vi "Elevator2.vi"() -> ()   [LabVIEW 2020]
uses:
  meter.ctl
  States.ctl
  <vilib>/MakerHub/LINX/Public/Peripherals/Digital/Digital Read N Chans.vi
  <vilib>/MakerHub/LINX/Private/Local IO/LinxDigitalRead.vi
  <vilib>/MakerHub/LINX/Public/Utilities/Check Channel.vi
  <vilib>/MakerHub/LINX/Public/Utilities/Open Serial.vi
  <vilib>/MakerHub/LINX/Private/Utilties/Generate Error.vi
  <vilib>/MakerHub/LINX/LMH-LINX.lvlib
panel:
  in  "Floor 1":bool
  in  "Floor 2":bool
  in  "Floor 3":bool
  in  "Floor 4":bool
  in  "DI Channels":u8[](array[numeric])
  in  "Serial Port":refnum<visa-resource-name>="N/A"
  in  "Run time error":errorcluster
  out "Arrow":u16(ring)
  out "Meter 1":T1 scale=1.0..4.0
  out "Meter 2":T1 scale=1.0..4.0
  out "Meter 4":T1 scale=1.0..4.0
  out "Meter 3":T1 scale=1.0..4.0
  in  "Down (2)":bool
  in  "Up (1)":bool
  in  "Up (2)":bool
  in  "Up (3)":bool
  in  "Down (3)":bool
  in  "Down (4)":bool
  out "Ring 1":u16(ring)
  out "Ring 2":u16(ring)
  out "Ring 3":u16(ring)
  out "Ring 4":u16(ring)
  out "Slider":dbl(slide) step=1.0 scale=1.0..4.0
  out "Floor #":u8
  in  "stop":bool
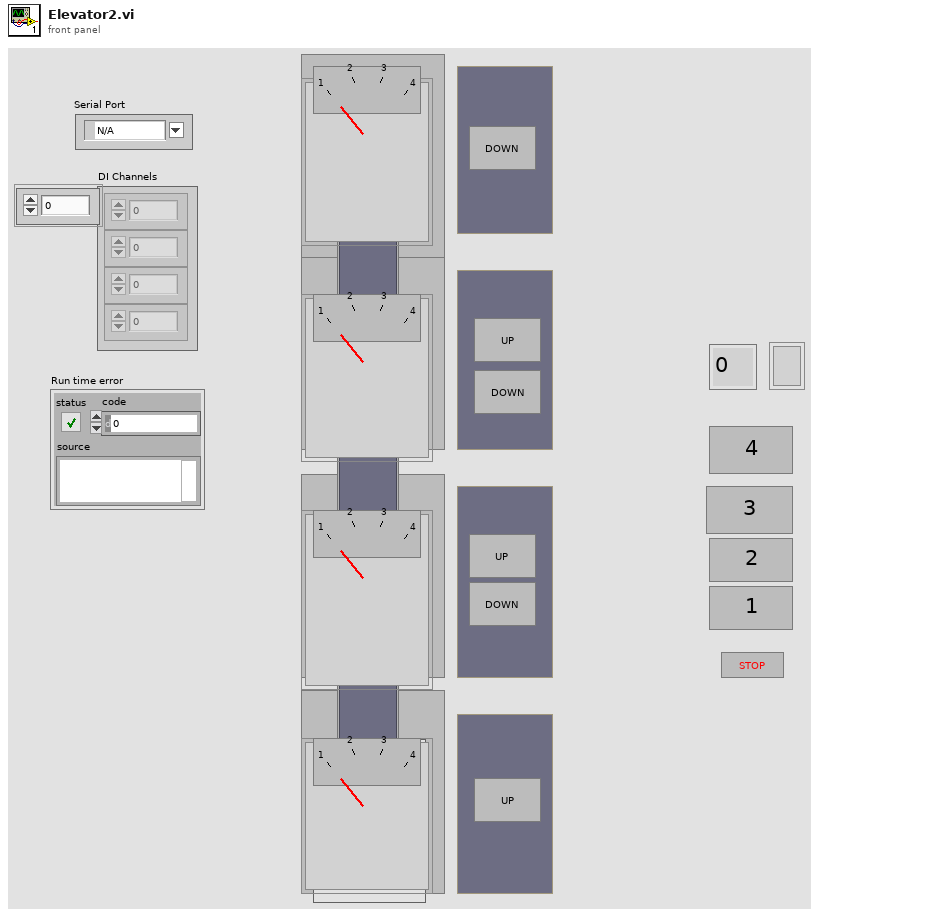
[diagram p1: front panel]
types:
  T1 = typedef "meter.ctl" = u16
  T2 = typedef "States.ctl" = enum16{"Initialization", "Check for Input", "Moving to 1", "Moving to 2", "Moving to 3", "Moving to 4", "Arrival"}
  T3 = typedef "LMH-LINX.lvlib/LINX Ref.ctl" = cluster{"IO":T4, "Interface":T5, "LINX Device Config":T6}
  T4 = typedef "LMH-LINX.lvlib/Platform.ctl" = enum16{"Remote", "Local"}
  T5 = typedef "LMH-LINX.lvlib/Interface.ctl" = enum16{"Serial", "TCP"}
  T6 = typedef "LMH-LINX.lvlib/Device.lvlib/LINX Device Config.ctl" = cluster{"Interface":T5, "COM Port":refnum<visa-resource-name>, "TCP Configuration":T7, "Device Family":u8, "Device ID":u8, "Device Name":string, "TCP Ref":refnum<k5>, "Channels":T8}
  T7 = typedef "LMH-LINX.lvlib/Device.lvlib/TCP Config.ctl" = cluster{"IP Address":string, "Port":u16}
  T8 = typedef "LMH-LINX.lvlib/Channels.ctl" = cluster{"DI":u8[], "DO":u8[], "AI":u8[], "AO":u8[], "PWM":u8[], "QE":u8[], "UART":u8[], "I2C 2":u8[], "SPI":u8[], "CAN":u8[], "Servo":u8[], "AI Ref (V)":dbl, "AI Resolution (Bits)":u8, "AO Ref (V)":dbl, "AO Resolution (Bits)":u8}
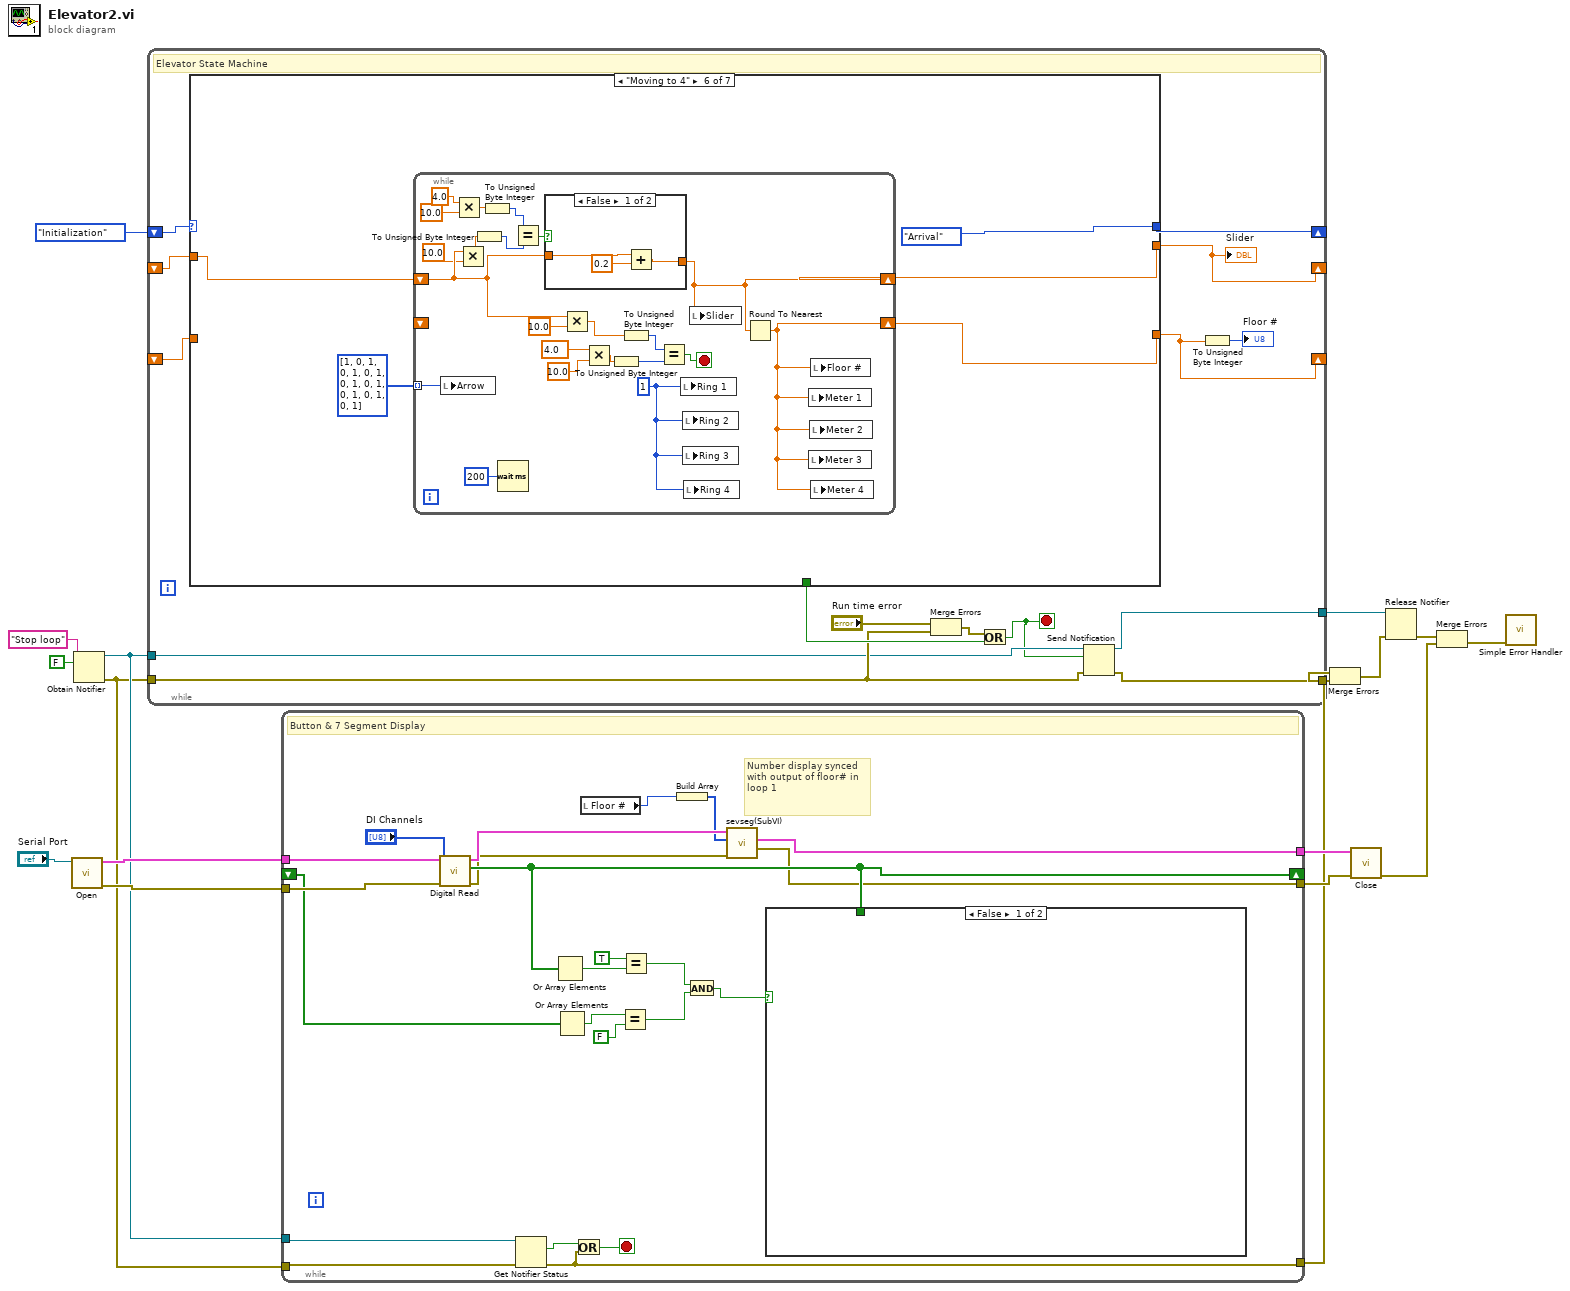
[diagram p0: block diagram]
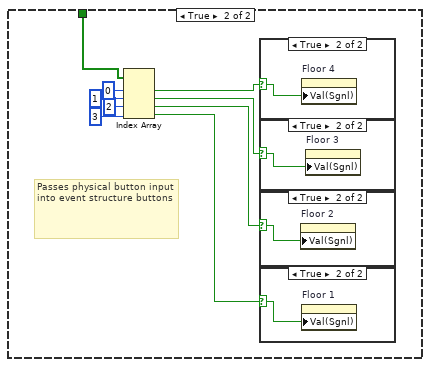
[diagram p2: hidden frame]
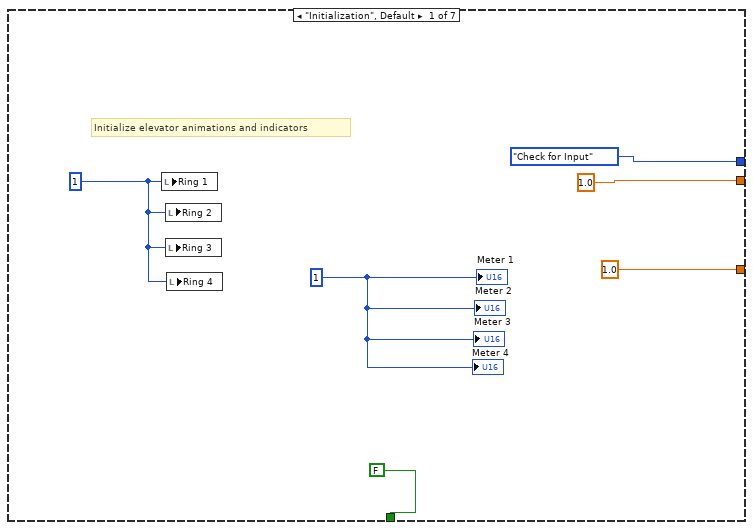
[diagram p7: hidden frame]
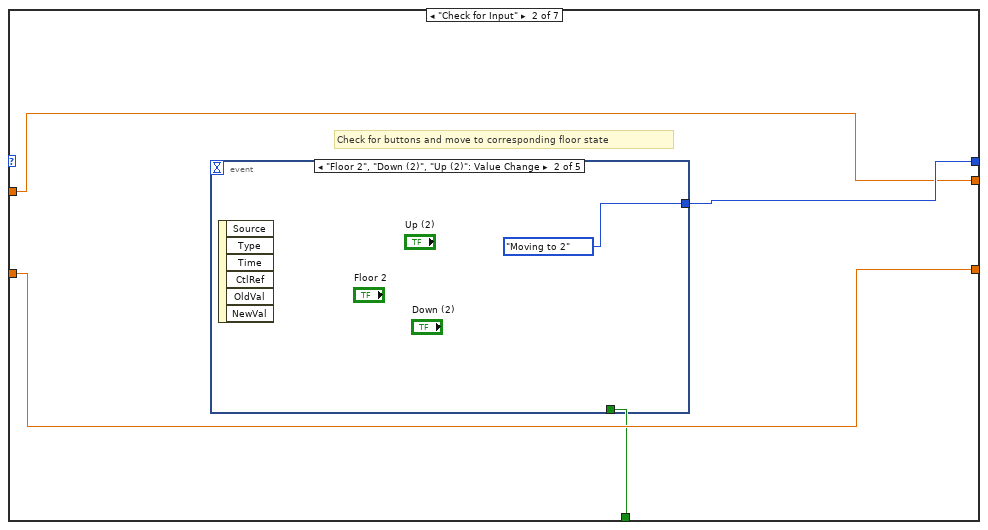
[diagram p8: hidden frame]
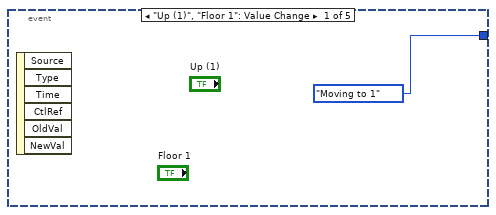
[diagram p9: hidden frame]
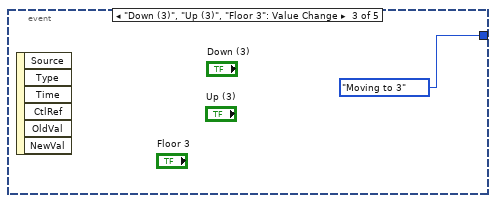
[diagram p10: hidden frame]
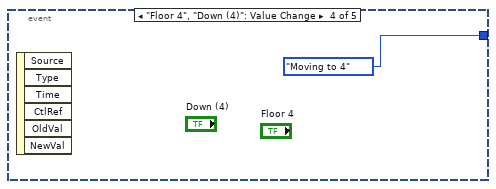
[diagram p11: hidden frame]
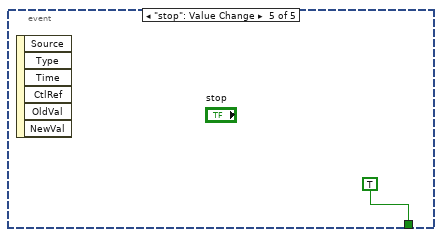
[diagram p12: hidden frame]
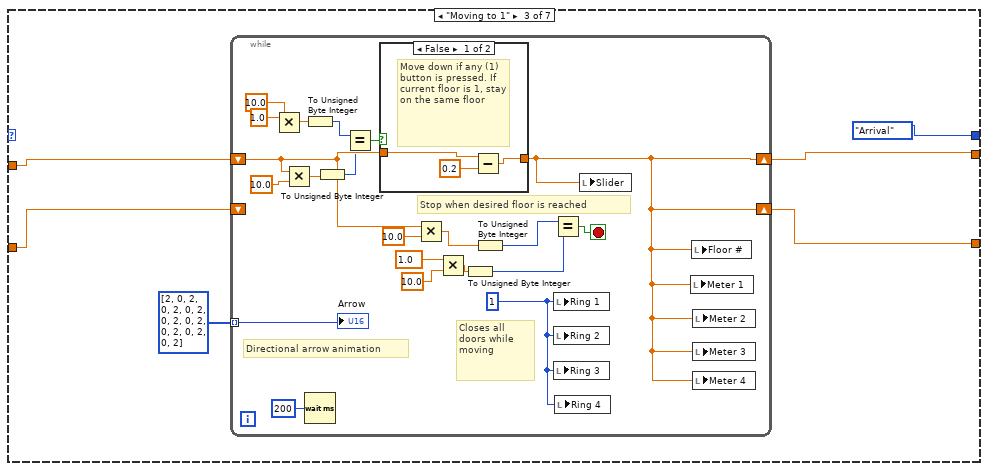
[diagram p13: hidden frame]
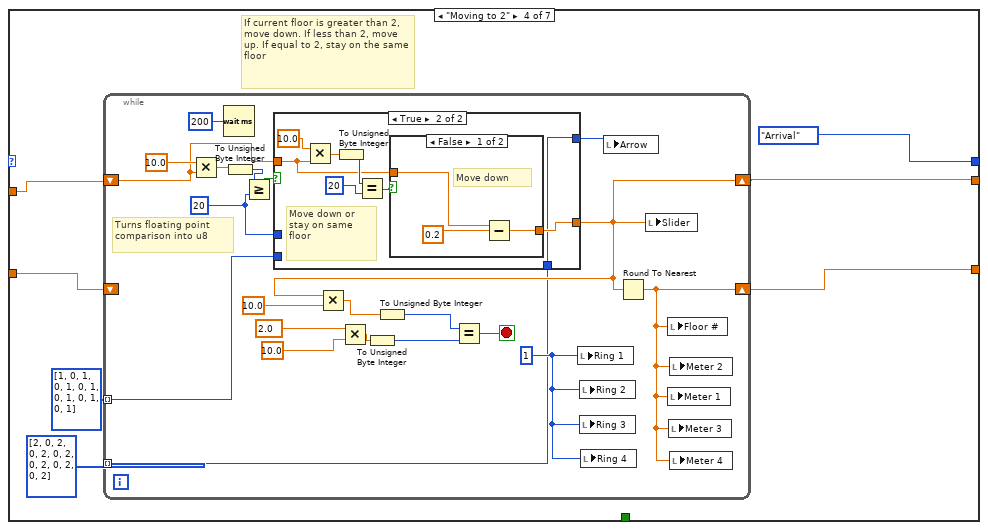
[diagram p15: hidden frame]
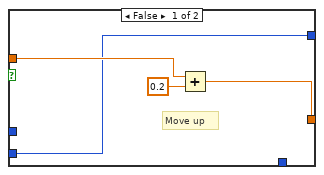
[diagram p16: hidden frame]
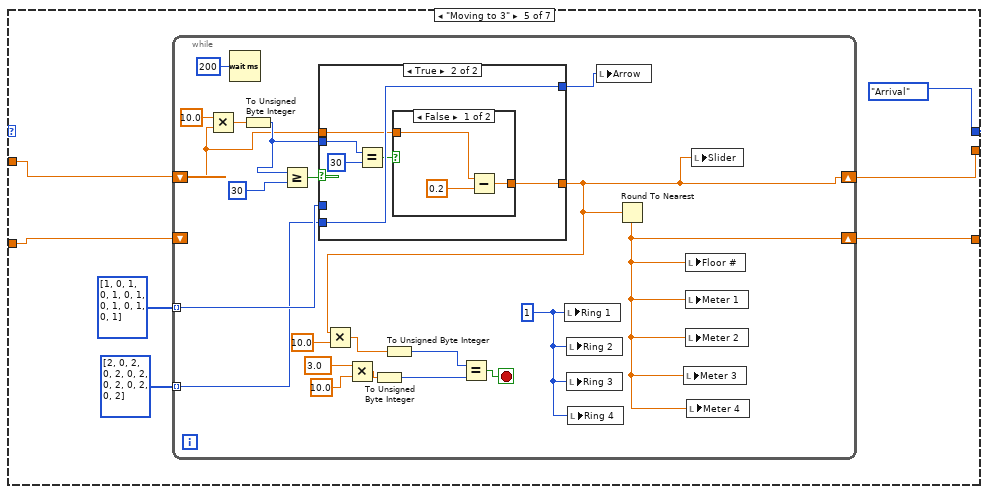
[diagram p18: hidden frame]
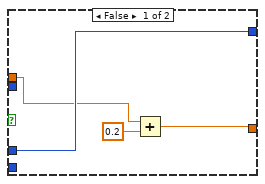
[diagram p19: hidden frame]
diagram:
  n1 = call-poly <vilib>:"Open.vi"("Serial Port"="Serial Port") -> ("Error Out"=w8:errorcluster, "LINX Resource"=w9:T3)  [unwired: 8 in, 1 out]
  n2 = Obtain Notifier(name (unnamed)="Stop loop", notification data type=FALSE) -> (notifier out=w4:refnum<notifier>, error out=w3:errorcluster)  [unwired: 2 in, 1 out]
  n3 = while {
    shift-right: [w31] -> _
    shift-left: States."Initialization" -> [w32]
    shift-right: [w27] -> _
    shift-left: _ -> [w29]
    shift-right: [w28] -> _
    shift-left: _ -> [w30]
    tunnel: w3 -> [w22]
    tunnel: w4 -> [w21]
    tunnel: [w19] -> w2
    tunnel: [w18] -> w14
    stop <- w20 stop-if-true
    # "Elevator State Machine"
    n4 = case shown="\"Moving to 4\"" w32 {
      tunnel: [1.0 ("Slider") w41 w51 w84 w127 w167 w202] -> w28
      tunnel: [1.0 ("Floor #") w40 w49 w81 w126 w166 w201] -> w27
      tunnel: [States."Check for Input" w42 States."Arrival" States."Arrival" States."Arrival" States."Arrival" States."Check for Input"] -> w31
      tunnel: w30 -> [_ w41 w52 w83 w128 w168 w202]
      tunnel: w29 -> [_ w40 w50 w82 w125 _ w201]
      tunnel: [FALSE w39 _ _ _ _ _] -> w23
      frame "Initialization", Default {
        w36 = T1 1 ("Meter 1")
        w37 = u16 1 ("Ring 1")
        # "Initialize elevator animations and indicators"
        n5 = local write "Ring 1"(w37) -> ()
        n6 = local write "Ring 2"(w37) -> ()
        n7 = local write "Ring 3"(w37) -> ()
        n8 = local write "Ring 4"(w37) -> ()
        "Meter 3" <- w36
        "Meter 2" <- w36
        "Meter 1" <- w36
        "Meter 4" <- w36
      }
      frame "Check for Input" {
        # "Check for buttons and move to corresponding floor state"
        n9 = event shown="[1] \"Floor 2\", \"Down (2)\", \"Up (2)\": Value Change" {
          selector: _ -> [_ _ _ _ _]
          dyn-events: _ -> [_ _ _ _ _]
          timeout: _ -> [_ _ _ _ _]
          tunnel: [States."Moving to 1" States."Moving to 2" States."Moving to 3" States."Moving to 4" _] -> w42
          tunnel: [_ _ _ _ TRUE] -> w39
          event "Up (1)", "Floor 1": Value Change {
            n10 = event-data() -> ()  [unwired: 1 in, 6 out]
          }
          event "Floor 2", "Down (2)", "Up (2)": Value Change {
            n11 = event-data() -> ()  [unwired: 1 in, 6 out]
          }
          event "Down (3)", "Up (3)", "Floor 3": Value Change {
            n12 = event-data() -> ()  [unwired: 1 in, 6 out]
          }
          event "Floor 4", "Down (4)": Value Change {
            n13 = event-data() -> ()  [unwired: 1 in, 6 out]
          }
          event "stop": Value Change {
            n14 = event-data() -> ()  [unwired: 1 in, 6 out]
          }
        }
      }
      frame "Moving to 1" {
        n15 = while {
          shift-right: [w55] -> w51
          shift-left: w52 -> [w63]
          shift-right: [w55] -> w49
          shift-left: w50 -> [_]
          tunnel: i32[] [2, 0, 2, 0, 2, 0, 2, 0, 2, 0, 2, 0, 2, 0, 2, 0, 2] -> [w54] mode=indexing
          stop <- w74 stop-if-true
          w65 = u16 1 ("Ring 1")
          # "Stop when desired floor is reached"
          # "Closes all doors while moving"
          # "Directional arrow animation"
          n16 = Multiply(x=1.0, y=10.0) -> (x*y=w56:dbl)
          n17 = Multiply(x=w63, y=10.0) -> (x*y=w62:dbl)
          n18 = To Unsigned Byte Integer(number=w56) -> (unsigned 8bit integer=w57:u8)
          n19 = Wait (ms)(milliseconds to wait=u32 200) -> ()  [unwired: 1 out]
          n20 = To Unsigned Byte Integer(number=w62) -> (unsigned 8bit integer=w60:u8)
          n21 = Equal?(x=w57, y=w60) -> (x = y?=w61:bool)
          n22 = case shown="False" w61 {
            tunnel: w63 -> [w76 w78]
            tunnel: [w75 w78] -> w55
            frame False {
              # "Move down if any (1) button is pressed. If current floor is 1, stay on the same floor"
              n23 = Subtract(x=w76, y=0.2) -> (x-y=w75:dbl)
            }
            frame True {
            }
          }
          n24 = Multiply(x=w63, y=10.0) -> (x*y=w67:dbl)
          n25 = Multiply(x=1.0 ("y"), y=10.0) -> (x*y=w69:dbl)
          n26 = To Unsigned Byte Integer(number=w69) -> (unsigned 8bit integer=w68:u8)
          n27 = To Unsigned Byte Integer(number=w67) -> (unsigned 8bit integer=w66:u8)
          n28 = Equal?(x=w66, y=w68) -> (x = y?=w74:bool)
          n29 = local write "Ring 1"(w65) -> ()
          n30 = local write "Ring 2"(w65) -> ()
          n31 = local write "Ring 3"(w65) -> ()
          n32 = local write "Ring 4"(w65) -> ()
          n33 = local write "Slider"(w55) -> ()
          n34 = local write "Meter 1"(w55) -> ()
          n35 = local write "Floor #"(w55) -> ()
          n36 = local write "Meter 2"(w55) -> ()
          n37 = local write "Meter 3"(w55) -> ()
          n38 = local write "Meter 4"(w55) -> ()
          "Arrow" <- w54
        }
      }
      frame "Moving to 2" {
        # "If current floor is greater than 2, move down. If less than 2, move up. If equal to 2, stay on the same floor"
        n39 = while {
          shift-right: [w96] -> w84
          shift-left: w83 -> [w88]
          shift-right: [w93] -> w81
          shift-left: w82 -> [_]
          tunnel: i32[] [1, 0, 1, 0, 1, 0, 1, 0, 1, 0, 1, 0, 1] -> [w92] mode=indexing
          tunnel: i32[] [2, 0, 2, 0, 2, 0, 2, 0, 2, 0, 2, 0, 2] -> [w90] mode=indexing
          stop <- w106 stop-if-true
          w95 = u16 1 ("Ring 1")
          w94 = u8 20 ("y")
          # "Turns floating point comparison into u8"
          n40 = Multiply(x=10.0, y=w88) -> (x*y=w86:dbl)
          n41 = Wait (ms)(milliseconds to wait=u32 200) -> ()  [unwired: 1 out]
          n42 = To Unsigned Byte Integer(number=w86) -> (unsigned 8bit integer=w87:u8)
          n43 = Greater Or Equal?(x=w87, y=w94) -> (x >= y?=w97:bool)
          n44 = case shown="True" w97 {
            tunnel: w88 -> [w109 w111]
            tunnel: [w108 w118] -> w96
            tunnel: w94 -> [_ _]
            tunnel: w92 -> [w107 _]
            tunnel: [w107 w117] -> w91
            tunnel: w90 -> [_ w117]
            frame False {
              # "Move up"
              n45 = Add(x=w109, y=0.2) -> (x+y=w108:dbl)
            }
            frame True {
              # "Move down or stay on same floor"
              n46 = Multiply(x=10.0, y=w111) -> (x*y=w112:dbl)
              n47 = To Unsigned Byte Integer(number=w112) -> (unsigned 8bit integer=w114:u8)
              n48 = Equal?(x=w114, y=u8 20) -> (x = y?=w116:bool)
              n49 = case shown="False" w116 {
                tunnel: [w121 w122] -> w118
                tunnel: w111 -> [w119 w122]
                frame False {
                  # "Move down"
                  n50 = Subtract(x=w119, y=0.2) -> (x-y=w121:dbl)
                }
                frame True {
                  # "Stay on the same floor"
                }
              }
            }
          }
          n51 = Multiply(x=w96, y=10.0) -> (x*y=w99:dbl)
          n52 = Multiply(x=2.0 ("y"), y=10.0) -> (x*y=w101:dbl)
          n53 = To Unsigned Byte Integer(number=w101) -> (unsigned 8bit integer=w100:u8)
          n54 = To Unsigned Byte Integer(number=w99) -> (unsigned 8bit integer=w98:u8)
          n55 = Equal?(x=w98, y=w100) -> (x = y?=w106:bool)
          n56 = local write "Ring 1"(w95) -> ()
          n57 = local write "Ring 2"(w95) -> ()
          n58 = local write "Ring 3"(w95) -> ()
          n59 = local write "Ring 4"(w95) -> ()
          n60 = local write "Arrow"(w91) -> ()
          n61 = Round To Nearest(number=w96) -> (nearest integer value=w93:dbl)
          n62 = local write "Slider"(w96) -> ()
          n63 = local write "Floor #"(w93) -> ()
          n64 = local write "Meter 1"(w93) -> ()
          n65 = local write "Meter 3"(w93) -> ()
          n66 = local write "Meter 2"(w93) -> ()
          n67 = local write "Meter 4"(w93) -> ()
        }
      }
      frame "Moving to 3" {
        n68 = while {
          shift-right: [w137] -> w127
          shift-left: w128 -> [w130]
          shift-right: [w138] -> w126
          shift-left: w125 -> [_]
          tunnel: i32[] [1, 0, 1, 0, 1, 0, 1, 0, 1, 0, 1, 0, 1] -> [w136] mode=indexing
          tunnel: i32[] [2, 0, 2, 0, 2, 0, 2, 0, 2, 0, 2, 0, 2] -> [w134] mode=indexing
          stop <- w150 stop-if-true
          w139 = u16 1 ("Ring 1")
          n69 = Multiply(x=10.0, y=w130) -> (x*y=w132:dbl)
          n70 = Wait (ms)(milliseconds to wait=u32 200) -> ()  [unwired: 1 out]
          n71 = To Unsigned Byte Integer(number=w132) -> (unsigned 8bit integer=w131:u8)
          n72 = Greater Or Equal?(x=w131, y=u8 30) -> (x >= y?=w141:bool)
          n73 = case shown="True" w141 {
            tunnel: [w153 w160] -> w137
            tunnel: w136 -> [w152 _]
            tunnel: [w152 w159] -> w135
            tunnel: w134 -> [_ w159]
            tunnel: w131 -> [_ w156]
            tunnel: w130 -> [w151 w155]
            frame False {
              n74 = Add(x=w151, y=0.2) -> (x+y=w153:dbl)
            }
            frame True {
              n75 = Equal?(x=w156, y=u8 30) -> (x = y?=w158:bool)
              n76 = case shown="False" w158 {
                tunnel: [w162 w164] -> w160
                tunnel: w155 -> [w161 w164]
                frame False {
                  n77 = Subtract(x=w161, y=0.2) -> (x-y=w162:dbl)
                }
                frame True {
                }
              }
            }
          }
          n78 = Multiply(x=w137, y=10.0) -> (x*y=w143:dbl)
          n79 = Multiply(x=3.0 ("y"), y=10.0) -> (x*y=w145:dbl)
          n80 = To Unsigned Byte Integer(number=w145) -> (unsigned 8bit integer=w144:u8)
          n81 = To Unsigned Byte Integer(number=w143) -> (unsigned 8bit integer=w142:u8)
          n82 = Equal?(x=w142, y=w144) -> (x = y?=w150:bool)
          n83 = local write "Ring 1"(w139) -> ()
          n84 = local write "Ring 2"(w139) -> ()
          n85 = local write "Ring 3"(w139) -> ()
          n86 = local write "Ring 4"(w139) -> ()
          n87 = local write "Arrow"(w135) -> ()
          n88 = Round To Nearest(number=w137) -> (nearest integer value=w138:dbl)
          n89 = local write "Meter 3"(w138) -> ()
          n90 = local write "Floor #"(w138) -> ()
          n91 = local write "Meter 1"(w138) -> ()
          n92 = local write "Meter 2"(w138) -> ()
          n93 = local write "Meter 4"(w138) -> ()
          n94 = local write "Slider"(w137) -> ()
        }
      }
      frame "Moving to 4" {
        n95 = while {
          shift-right: [w182] -> w167
          shift-left: w168 -> [w177]
          shift-right: [w171] -> w166
          shift-left: _ -> [_]
          tunnel: i32[] [1, 0, 1, 0, 1, 0, 1, 0, 1, 0, 1, 0, 1, 0, 1, 0, 1] -> [w170] mode=indexing
          stop <- w191 stop-if-true
          w181 = u16 1 ("Ring 1")
          n96 = local write "Arrow"(w170) -> ()
          n97 = Multiply(x=4.0 ("y"), y=10.0) -> (x*y=w173:dbl)
          n98 = Multiply(x=w177, y=10.0) -> (x*y=w175:dbl)
          n99 = To Unsigned Byte Integer(number=w175) -> (unsigned 8bit integer=w174:u8)
          n100 = To Unsigned Byte Integer(number=w173) -> (unsigned 8bit integer=w172:u8)
          n101 = Wait (ms)(milliseconds to wait=u32 200) -> ()  [unwired: 1 out]
          n102 = Equal?(x=w172, y=w174) -> (x = y?=w180:bool)
          n103 = case shown="False" w180 {
            tunnel: w177 -> [w194 w195]
            tunnel: [w192 w195] -> w182
            frame False {
              n104 = Add(x=w194, y=0.2) -> (x+y=w192:dbl)
            }
            frame True {
            }
          }
          n105 = Multiply(x=w177, y=10.0) -> (x*y=w184:dbl)
          n106 = Multiply(x=4.0 ("y"), y=10.0) -> (x*y=w186:dbl)
          n107 = To Unsigned Byte Integer(number=w186) -> (unsigned 8bit integer=w185:u8)
          n108 = To Unsigned Byte Integer(number=w184) -> (unsigned 8bit integer=w183:u8)
          n109 = Equal?(x=w183, y=w185) -> (x = y?=w191:bool)
          n110 = local write "Ring 1"(w181) -> ()
          n111 = local write "Ring 2"(w181) -> ()
          n112 = local write "Ring 3"(w181) -> ()
          n113 = local write "Ring 4"(w181) -> ()
          n114 = local write "Slider"(w182) -> ()
          n115 = Round To Nearest(number=w182) -> (nearest integer value=w171:dbl)
          n116 = local write "Meter 1"(w171) -> ()
          n117 = local write "Meter 3"(w171) -> ()
          n118 = local write "Meter 2"(w171) -> ()
          n119 = local write "Floor #"(w171) -> ()
          n120 = local write "Meter 4"(w171) -> ()
        }
      }
      frame "Arrival" {
        w196 = FALSE ("Floor 1")
        # "Reset buttons"
        n121 = case shown="1, Default" w202 {
          tunnel: [u16 0 ("Ring 1") u16 1 ("Ring 1") u16 1 ("Ring 1") u16 1 ("Ring 1")] -> w197
          tunnel: [u16 1 ("Ring 2") u16 0 ("Ring 2") u16 1 ("Ring 2") u16 1 ("Ring 2")] -> w198
          tunnel: [u16 1 ("Ring 3") u16 1 ("Ring 3") u16 0 ("Ring 3") u16 1 ("Ring 3")] -> w199
          tunnel: [u16 1 ("Ring 4") u16 1 ("Ring 4") u16 1 ("Ring 4") u16 0 ("Ring 4")] -> w200
          frame 1, Default {
            # "Open door based which floor is reached"
          }
          frame 2 {
          }
          frame 3 {
          }
          frame 4 {
          }
        }
        "Ring 1" <- w197
        "Ring 2" <- w198
        "Ring 3" <- w199
        "Ring 4" <- w200
        n122 = local write "Floor 3"(w196) -> ()
        n123 = local write "Floor 1"(w196) -> ()
        n124 = local write "Floor 4"(w196) -> ()
        n125 = local write "Floor 2"(w196) -> ()
      }
    }
    "Slider" <- w28
    n126 = Merge Errors("Run time error", w22) -> (w24:errorcluster)
    n127 = Or(x=w24, y=w23) -> (x .or. y?=w20:bool)
    n128 = Send Notification(notification=w20, notifier=w21, error in (no error)=w22) -> (notifier out=w18:refnum<notifier>, error out=w19:errorcluster)
    n129 = To Unsigned Byte Integer(number=w27) -> (unsigned 8bit integer=→"Floor #":u8)
  }
  n130 = while {
    tunnel: w9 -> [w242]
    tunnel: w8 -> [w241]
    tunnel: [w224] -> w7
    tunnel: [w222] -> w6
    shift-right: [w231] -> _
    shift-left: _ -> [w235]
    tunnel: w4 -> [w230]
    tunnel: w3 -> [w229]
    tunnel: [w226] -> w1
    stop <- w227 stop-if-true
    # "Number display synced with output of floor# in loop 1"
    # "Button & 7 Segment Display"
    n131 = call-poly <vilib>:"Digital Read.vi"("Error In"=w241, "DI Channels"="DI Channels", "LINX Resource"=w242) -> ("Error Out"=w223:errorcluster, "Values"=w231:bool[], "LINX Resource"=w225:T3)  [unwired: 6 in]
    n132 = Get Notifier Status(notifier=w230, error in (no error)=w229) -> (current notification=w228:bool, error out=w226:errorcluster)  [unwired: 3 out]
    n133 = Or Array Elements(Boolean array=w231) -> (logical OR=w239:bool)
    n134 = Or Array Elements(Boolean array=w235) -> (logical OR=w237:bool)
    n135 = Or(x=w228, y=w226) -> (x .or. y?=w227:bool)
    n136 = local read "Floor #"() -> (w221:u8)
    n137 = Equal?(x=w237, y=FALSE) -> (x = y?=w233:bool)
    n138 = Equal?(x=TRUE, y=w239) -> (x = y?=w234:bool)
    n139 = Build Array(w221) -> (w220:u8[])
    n140 = And(x=w234, y=w233) -> (x .and. y?=w232:bool)
    n141 = call "sevseg(SubVI).vi"("error in (no error)"=w223, "Data"=w220, "LINX Resource in"=w225) -> ("error out"=w222:errorcluster, "LINX Resource out"=w224:T3)  [unwired: 6 in, 1 out]
    n142 = case shown="False" w232 {
      tunnel: w231 -> [_ w247]
      frame False {
      }
      frame True {
        # "Passes physical button input into event structure buttons"
        n143 = Index Array(array=w247, index #1=0 ("index"), index #2=1 ("index"), index #3=2 ("index"), index #4=3 ("index")) -> (element #1=w246:bool, element #2=w245:bool, element #3=w244:bool, element #4=w243:bool)
        n144 = case shown="True" w246 {
          selector: w246 -> [_ w255]
          frame False {
          }
          frame True {
            n145 = property on="Floor 4" class="Bool (strict)"("Val(Sgnl)"=w255) -> ()  [unwired: 2 in, 2 out]
          }
        }
        n146 = case shown="True" w245 {
          selector: w245 -> [_ w254]
          frame False {
          }
          frame True {
            n147 = property on="Floor 3" class="Bool (strict)"("Val(Sgnl)"=w254) -> ()  [unwired: 2 in, 2 out]
          }
        }
        n148 = case shown="True" w244 {
          selector: w244 -> [_ w253]
          frame False {
          }
          frame True {
            n149 = property on="Floor 2" class="Bool (strict)"("Val(Sgnl)"=w253) -> ()  [unwired: 2 in, 2 out]
          }
        }
        n150 = case shown="True" w243 {
          selector: w243 -> [_ w252]
          frame False {
          }
          frame True {
            n151 = property on="Floor 1" class="Bool (strict)"("Val(Sgnl)"=w252) -> ()  [unwired: 2 in, 2 out]
          }
        }
      }
    }
  }
  n152 = Merge Errors(w2, w1) -> (w13:errorcluster)
  n153 = call <vilib>:"Close.vi"("Error In"=w6, "LINX Resource"=w7) -> ("Error Out"=w5:errorcluster)  [unwired: 9 in]
  n154 = Release Notifier(notifier=w14, error in (no error)=w13) -> (error out=w12:errorcluster)  [unwired: 1 in, 2 out]
  n155 = Merge Errors(w12, w5) -> (w11:errorcluster)
  n156 = call <vilib>:"Simple Error Handler.vi"("error in (no error)"=w11) -> ()  [unwired: 4 in, 5 out]
